vi "AssertsEqual.vi"(0 "VI Reference In":refnum<vi>, 1 "Label (VI Title)":string="Default", 11 "error in (no error)":errorcluster) -> (4 "VI Reference Out":refnum<vi>, 15 "error out":errorcluster)   [LabVIEW 2016, in "DronaTest.lvlib"]
uses:
  DronaTest.lvlib
  main/apis/Stimulus/KeyBoardSimulation/ValueSignalLatchBooleanString.vi
  main/apis/Assert/AssertControlValue/Equal.vi
  <vilib>/addons/_JKI Toolkits/Caraya/classes/Assert/Assert Not Error.vi
  <vilib>/addons/_JKI Toolkits/Caraya/classes/Assert/Assert Error.vi
  <vilib>/addons/_JKI Toolkits/Caraya/classes/Test/Test.lvclass
  main/Drona.lvlib
  <vilib>/addons/_JKI Toolkits/Caraya/classes/Assert/Assert.lvclass
  main/apis/Stimulus/KeyBoardSimulation/KeyboardSimulation.lvlib
  main/apis/Assert/AssertControlValue/AssertControlValue.lvlib
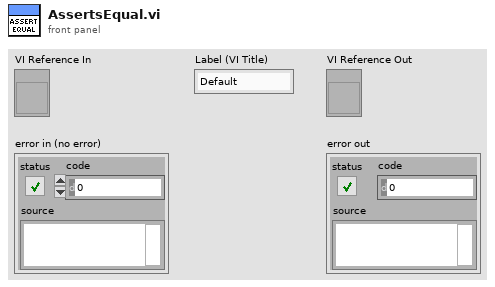
[diagram p1: front panel]
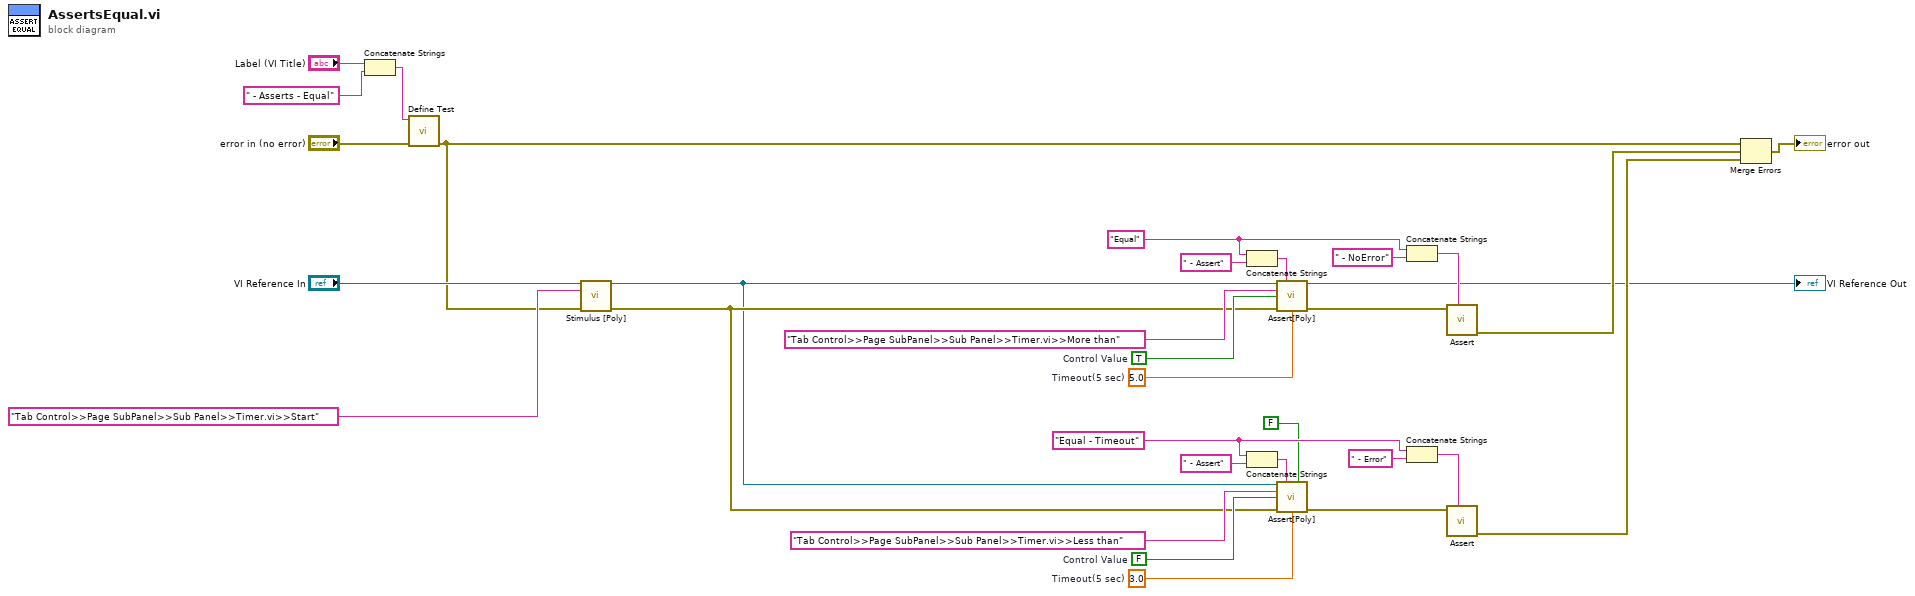
[diagram p0: block diagram]
diagram:
  w24 = FALSE  # Control Value
  w14 = 3.0  # Timeout(5 sec)
  w13 = "Equal - Timeout" ("string")
  w15 = 5.0  # Timeout(5 sec)
  w16 = TRUE  # Control Value
  w17 = "Equal" ("string")
  n1 = Concatenate Strings("Label (VI Title)", " - Asserts - Equal" ("Label (VI Title)")) -> (w28:string)
  n2 = call <vilib>:"Define Test.vi"("error in (no error)"="error in (no error)", "Label (VI Title)"=w28) -> ("error out"=w25:errorcluster)  [unwired: 9 in]
  n3 = call-poly "Stimulus [Poly].vi"("VI Reference In"="VI Reference In", "Control Path"="Tab Control>>Page SubPanel>>Sub Panel>>Timer.vi>>Start", "error in"=w25) -> ("VI Reference Out"=w4:refnum<vi>, "error out"=w5:errorcluster)  [unwired: 11 in]
  n4 = Concatenate Strings(w17, " - Assert" ("string")) -> (w19:string)
  n5 = Concatenate Strings(w13, " - Assert" ("string")) -> (w11:string)
  n6 = call-poly "Assert[Poly].vi"("VI Reference In"=w4, "Label"=w19, "Control Path"="Tab Control>>Page SubPanel>>Sub Panel>>Timer.vi>>More than", "Control Value"=w16, "Error In"=w5, "Timeout(5 sec)"=w15) -> ("VI Reference Out"=→"VI Reference Out":refnum<vi>, "Error Out"=w20:errorcluster)  [unwired: 8 in]
  n7 = call-poly "Assert[Poly].vi"("VI Reference In"=w4, "Label"=w11, "Assert Only? (F)"=FALSE, "Control Path"="Tab Control>>Page SubPanel>>Sub Panel>>Timer.vi>>Less than", "Control Value"=w24, "Error In"=w5, "Timeout(5 sec)"=w14) -> ("Error Out"=w10:errorcluster)  [unwired: 7 in, 1 out]
  n8 = Concatenate Strings(w17, " - NoError" ("string")) -> (w18:string)
  n9 = Concatenate Strings(w13, " - Error" ("string")) -> (w12:string)
  n10 = call-poly <vilib>:"Assert.vi"("Label"=w18, "Not Error?"=w20) -> ("error out"=w3:errorcluster)  [unwired: 9 in]
  n11 = call-poly <vilib>:"Assert.vi"("Label"=w12, "Error?"=w10) -> ("error out"=w2:errorcluster)  [unwired: 9 in]
  n12 = Merge Errors(w25, w3, w2) -> (→"error out":errorcluster)
